vi "PH_Powermeter_BaseClass.set current Settings.vi"(0 "VI in":refnum<vi>, 2 "Current Settings":T1, 5 "error in (no error)":errorcluster) -> (14 "VI out":refnum<vi>, 19 "error out":errorcluster)   [LabVIEW 2014, in "PH_Powermeter_BaseClass.lvlib"]
uses:
  PH_Powermeter_BaseClass.lvlib
  PH_gentec_BaseClass.Head Settings.ctl
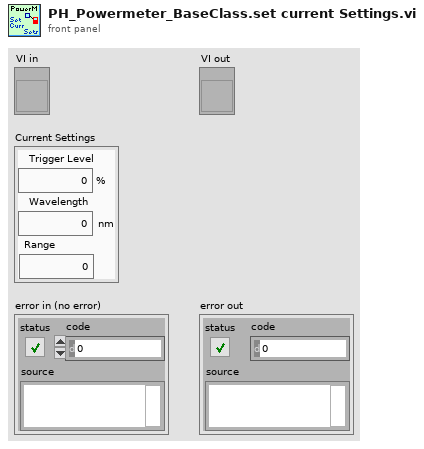
[diagram p1: front panel]
types:
  T1 = typedef "PH_Powermeter_BaseClass.lvlib/PH_gentec_BaseClass.Head Settings.ctl" = cluster{"Trigger Level":dbl, "Wavelength":u32, "Range":u32}
  T2 = typedef "PH_Powermeter_BaseClass.lvlib/PH_Powermeter_BaseClass.i attribute.ctl" = cluster{"GUI References":T3, "Connection":T4, "Head Attributes":T6, "VISA resource":refnum<visa-resource-name>, "Energy":T7, "Service ID Energy":i32, "Wanted Settings":T1, "Current Settings":T1}
  T3 = typedef "PH_Powermeter_BaseClass.lvlib/PH_Powermeter_BaseClass.GUI Refs.ctl" = cluster{"Head Attributes":refnum<vi>, "Energy":refnum<vi>, "Connection":refnum<vi>, "VISA Resource":refnum<vi>, "Scaling Factor":refnum<vi>, "Range":refnum<vi>, "Wavelength":refnum<vi>, "Trigger Level":refnum<vi>, "Wanted Settings":refnum<vi>, "Current Settings":refnum<vi>}
  T4 = typedef "PH_Powermeter_BaseClass.lvlib/PH_Powermeter_BaseClass.Connection.ctl" = cluster{"failed checks":i8, "Timeout":bool, "Data read":string, "Failure":bool, "Error":bool, "State":T5}
  T5 = typedef "PH_Powermeter_BaseClass.lvlib/PH_Powermeter_BaseClass.State.ctl" = enum32{"off", "operating", "opened", "checked", "connected", "Sets to change", "running"}
  T6 = typedef "PH_Powermeter_BaseClass.lvlib/PH_Powermeter_BaseClass.Head Attributes.ctl" = cluster{"Instrument Type":string, "Head Version":string, "Head Name":string, "Serial Number":string, "Firmware":string, "Sensor Type":string, "MinimumRange":u32, "Maximum Range":u32, "Min Wavelength":i32, "Max Wavelength":i32}
  T7 = typedef "PH_Powermeter_BaseClass.lvlib/PH_Powermeter_BaseClass.Energy.ctl" = cluster{"current Value":dbl, "unscaled":dbl, "Scaling Factor":dbl}
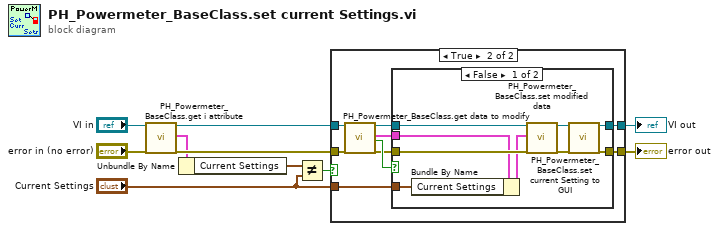
[diagram p0: block diagram]
diagram:
  n1 = call "PH_Powermeter_BaseClass.get i attribute.vi"("i ref in"="VI in", "error in (no error)"="error in (no error)") -> ("i ref out"=w5:refnum<vi>, "i attribute"=w4:T2, "error out"=w7:errorcluster)  [unwired: 15 in]
  n2 = Unbundle By Name(w4) -> ("Current Settings"=w3:T1)
  n3 = Not Equal?(x=w3, y="Current Settings") -> (x != y?=w1:bool)
  n4 = case shown="True" w1 {
    tunnel: [w12 w19] -> w10
    tunnel: [w11 w17] -> w9
    tunnel: w7 -> [w11 w15]
    tunnel: w5 -> [w12 w14]
    tunnel: "Current Settings" -> [_ w13]
    frame False {
    }
    frame True {
      n5 = call "PH_Powermeter_BaseClass.get data to modify.vi"("i ref in"=w14, "error in (no error)"=w15) -> ("i ref out"=w18:refnum<vi>, "i attribute"=w20:T2, "timed out"=w21:bool, "error out"=w16:errorcluster)  [unwired: 14 in]
      n6 = case shown="False" w21 {
        tunnel: w16 -> [w30 w31]
        tunnel: [w24 w31] -> w17
        tunnel: w18 -> [w28 w32]
        tunnel: [w22 w32] -> w19
        tunnel: w20 -> [w27 _]
        tunnel: w13 -> [w25 _]
        frame False {
          n7 = Bundle By Name(cluster=w27, "Current Settings"=w25) -> (w26:T2)
          n8 = call "PH_Powermeter_BaseClass.set modified data.vi"("i ref in"=w28, "i attribute"=w26, "error in (no error)"=w30) -> ("i ref out"=w23:refnum<vi>, "error out"=w29:errorcluster)  [unwired: 15 in]
          n9 = call "PH_Powermeter_BaseClass.set current Setting to GUI.vi"("VI in"=w23, "error in (no error)"=w29) -> ("VI out"=w22:refnum<vi>, "error out"=w24:errorcluster)  [unwired: 16 in]
        }
        frame True {
        }
      }
    }
  }
  "VI out" <- w10
  "error out" <- w9
